vi "rotateAroundModule.vi"(9 "module":u16(ring) items=["Front Left", "Front Right", "Back Left", "Back RIght"], 10 "rotation":dbl) -> ()   [LabVIEW 2020]
uses:
  <vilib>/Rock Robotics/WPI/ThirdParty/REV Robotics/REVLib/Typedef/Spark MAX Control Type.ctl
  <vilib>/Rock Robotics/WPI/ThirdParty/Sensors/navX/_TypeDefs/FRIC_navX_DeviceNumbersTypeDef.ctl
  Robot Global Data.vi
panel:
  # "handy dandy table"
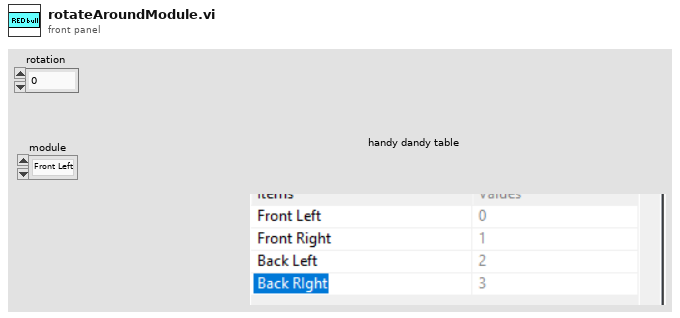
[diagram p1: front panel]
types:
  T1 = typedef "FRIC_navX_DeviceNumbersTypeDef.ctl" = enum16{"Dev0", "Dev1", "Dev2", "Dev3"}
  T2 = typedef "Spark MAX Control Type.ctl" = enum16{"Percent VBus", "Voltage", "Velocity", "Position", "Smart Motion", "Current", "Smart Velocity"}
  T3 = cluster{"Yaw":dbl, "Roll":dbl, "Pitch":dbl, "Heading":dbl, "Fused Heading":dbl}
  T4 = cluster{"FL":cluster{"proportional gain (Kc)":dbl, "integral time (Ti, min)":dbl, "derivative time (Td, min)":dbl}, "FR":cluster{"proportional gain (Kc)":dbl, "integral time (Ti, min)":dbl, "derivative time (Td, min)":dbl}, "BL":cluster{"proportional gain (Kc)":dbl, "integral time (Ti, min)":dbl, "derivative time (Td, min)":dbl}, "BR":cluster{"proportional gain (Kc)":dbl, "integral time (Ti, min)":dbl, "derivative time (Td, min)":dbl}}
  T5 = typedef "WPI_MotorControlDeviceRef.ctl" = cluster{"DeviceStatus":errorcluster, "Type":T6, "PWM":cluster{"PWM Channel":T7, "DeadBand":T8}, "CAN":cluster{"Device Number":u8, "SetOutput VI Ref":variant, "GetOutput VI Ref":variant, "Enable VI Ref":variant, "Disable VI Ref":variant, "Data":variant}, "Invert":bool, "DIO PWM":cluster{"PWM \"Enable\" Channel":T7, "DIOChannel":T9, "PWM Rate":dbl}}
  T6 = typedef "WPI_MotorControlType.ctl" = enum16{"PWM", "CAN", "DIO PWM"}
  T7 = typedef "FPGA_DIOPWMChannel.ctl" = enum8{"PWM 0", "PWM 1", "PWM 2", "PWM 3", "PWM 4", "PWM 5", "PWM 6", "PWM 7", "PWM 8", "PWM 9", "PWM MXP 0", "PWM MXP 1", "PWM MXP 2", "PWM MXP 3", "PWM MXP 4", "PWM MXP 5", "PWM MXP 6", "PWM MXP 7", "PWM MXP 8", "PWM MXP 9", "Invalid"}
  T8 = typedef "WPI_PWMDeadband.ctl" = cluster{"Name":string, "maxPositivePwm":i32, "minPositivePwm":i32, "centerPwm":i32, "maxNegativePwm":i32, "minNegativePwm":i32, "angularRange":u16}
  T9 = typedef "FPGA_DIOChannel.ctl" = enum8{"DIO 0", "DIO 1", "DIO 2", "DIO 3", "DIO 4", "DIO 5", "DIO 6", "DIO 7", "DIO 8", "DIO 9", "DIO MXP 0", "DIO MXP 1", "DIO MXP 2", "DIO MXP 3", "DIO MXP 4", "DIO MXP 5", "DIO MXP 6", "DIO MXP 7", "DIO MXP 8", "DIO MXP 9", "DIO MXP 10", "DIO MXP 11", "DIO MXP 12", "DIO MXP 13", "DIO MXP 14", "DIO MXP 15", "SPI Port CS1", "SPI Port CS2", "SPI Port CS3", "SPI Port MISO", "SPI Port MOSI", "Invalid"}
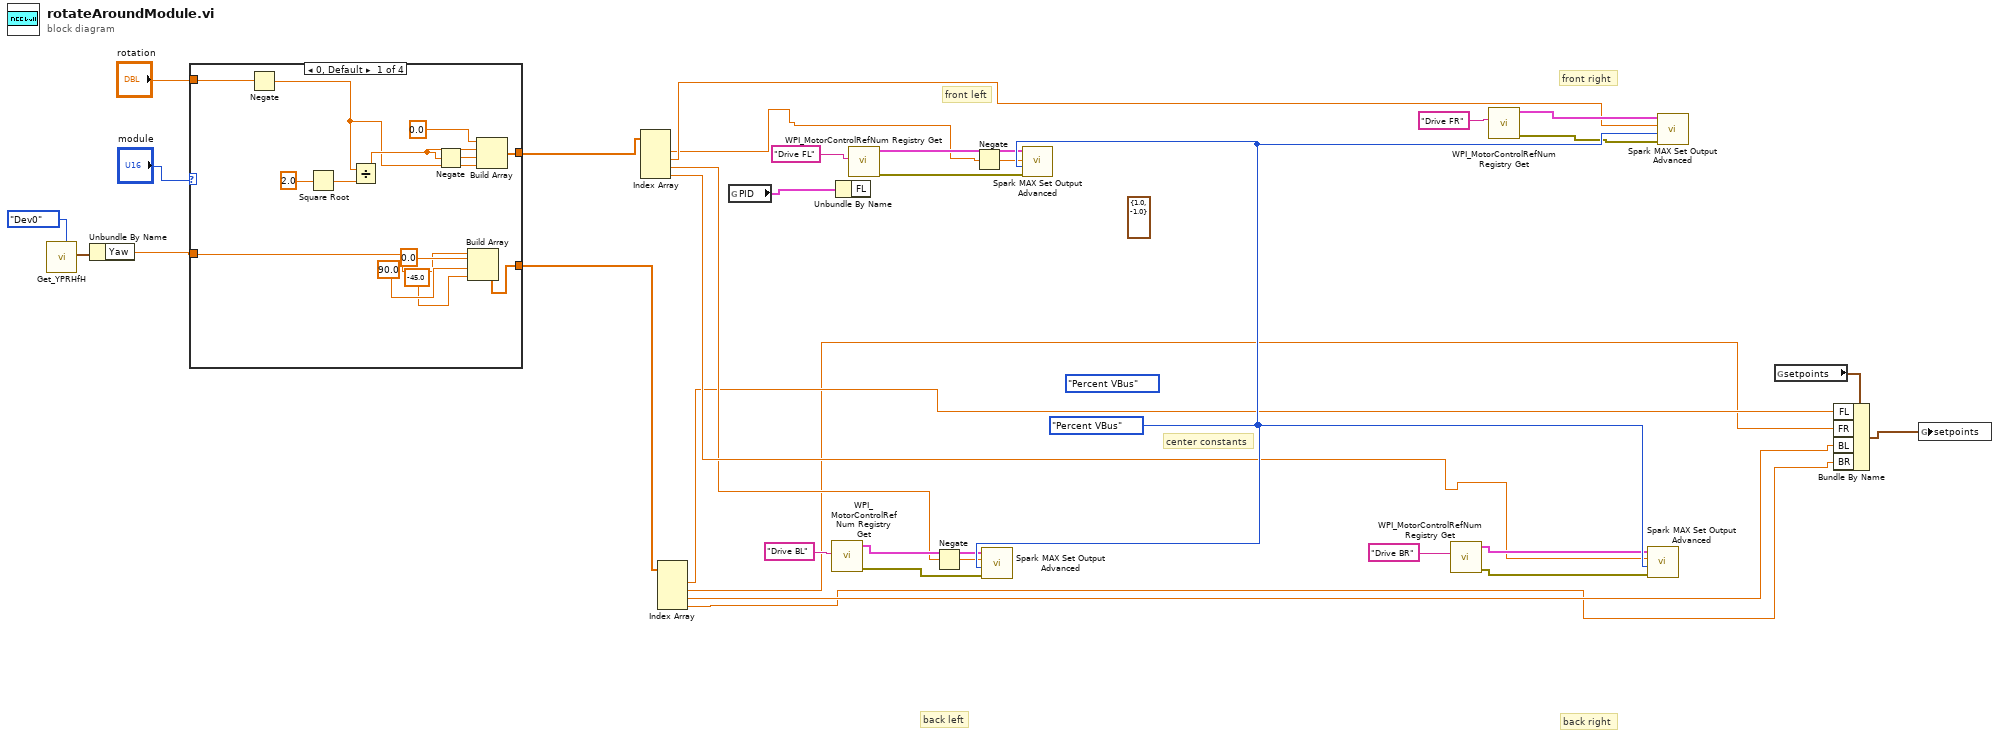
[diagram p0: block diagram]
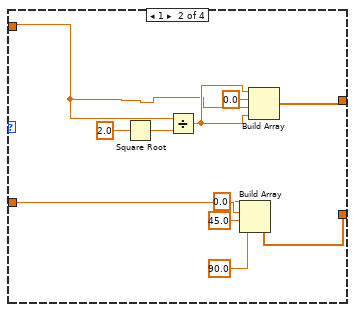
[diagram p2: hidden frame]
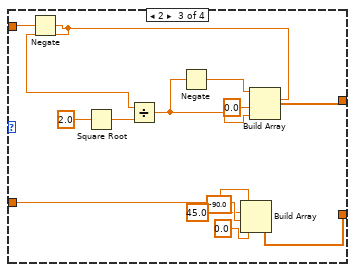
[diagram p3: hidden frame]
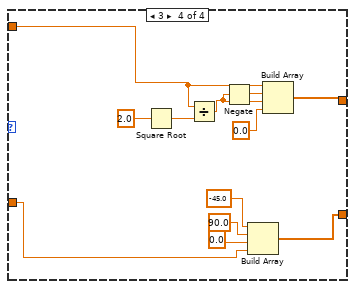
[diagram p4: hidden frame]
diagram:
  w28 = Spark_MAX_Control_Type."Percent VBus" ("Control Mode")
  (unwired) Spark_MAX_Control_Type."Percent VBus" ("Control Mode")
  (unwired) cluster{"output high":dbl, "output low":dbl} {"output high"=1.0, "output low"=-1.0} ("output range")
  # "center constants"
  # "back right"
  # "back left"
  # "front right"
  # "front left"
  n1 = call <vilib>:"Get_YPRHfH.vi"("Device Number"=FRIC_navX_DeviceNumbersTypeDef."Dev0") -> ("YRPHfH"=w12:T3)  [unwired: 10 in]
  n2 = Unbundle By Name(w12) -> ("Yaw"=w7:dbl)
  n3 = case shown="0, Default" "module" {
    tunnel: "rotation" -> [w35 w47 w58 w76]
    tunnel: [w43 w57 w70 w79] -> w17
    tunnel: [w42 w56 w69 w80] -> w14
    tunnel: w7 -> [w38 w55 w68 w81]
    frame 0, Default {
      n4 = Negate(x=w35) -> (-x=w34:dbl)
      n5 = Square Root(x=2.0) -> (sqrt(x)=w45:dbl)
      n6 = Divide(x=w34, y=w45) -> (x/y=w36:dbl)
      n7 = Negate(x=w36) -> (-x=w37:dbl)
      n8 = Build Array(w38, 0.0 ("element"), 90.0 ("element"), -45.0 ("element")) -> (w42:dbl[])
      n9 = Build Array(0.0, w36, w37, w34) -> (w43:dbl[])
    }
    frame 1 {
      n10 = Square Root(x=2.0) -> (sqrt(x)=w53:dbl)
      n11 = Divide(x=w47, y=w53) -> (x/y=w52:dbl)
      n12 = Build Array(0.0 ("element"), w55, 45.0 ("element"), 90.0 ("element")) -> (w56:dbl[])
      n13 = Build Array(w52, 0.0 ("element"), w47, w52) -> (w57:dbl[])
    }
    frame 2 {
      n14 = Negate(x=w58) -> (-x=w59:dbl)
      n15 = Square Root(x=2.0) -> (sqrt(x)=w66:dbl)
      n16 = Divide(x=w59, y=w66) -> (x/y=w61:dbl)
      n17 = Negate(x=w61) -> (-x=w60:dbl)
      n18 = Build Array(-90.0 ("element"), 45.0 ("element"), w68, 0.0 ("element")) -> (w69:dbl[])
      n19 = Build Array(w60, w59, 0.0 ("element"), w61) -> (w70:dbl[])
    }
    frame 3 {
      n20 = Square Root(x=2.0) -> (sqrt(x)=w78:dbl)
      n21 = Divide(x=w76, y=w78) -> (x/y=w71:dbl)
      n22 = Negate(x=w71) -> (-x=w72:dbl)
      n23 = Build Array(-45.0 ("element"), 90.0 ("element"), 0.0 ("element"), w81) -> (w80:dbl[])
      n24 = Build Array(w76, w72, w71, 0.0 ("element")) -> (w79:dbl[])
    }
  }
  n25 = Index Array(array=w17) -> (element #1=w11:dbl, element #2=w16:dbl, element #3=w9:dbl, element #4=w15:dbl)  [unwired: 4 in]
  n26 = Index Array(array=w14) -> (element #1=w4:dbl, element #2=w3:dbl, element #3=w2:dbl, element #4=w1:dbl)  [unwired: 4 in]
  n27 = global read "Robot Global Data.vi" "PID"() -> (w19:T4)
  n28 = call <vilib>:"WPI_MotorControlRefNum Registry Get.vi"("refnum name"="Drive BL") -> ("error out"=w26:errorcluster, "MotorControlDevRef"=w27:T5)  [unwired: 9 in]
  n29 = Unbundle By Name(w19) -> ()  [unwired: 1 out]
  n30 = call <vilib>:"WPI_MotorControlRefNum Registry Get.vi"("refnum name"="Drive FL") -> ("error out"=w24:errorcluster, "MotorControlDevRef"=w25:T5)  [unwired: 9 in]
  n31 = Negate(x=w9) -> (-x=w8:dbl)
  n32 = Negate(x=w11) -> (-x=w10:dbl)
  n33 = call <vilib>:"Spark MAX Set Output Advanced.vi"("error in (no error)"=w26, "Control Mode"=w28, "Setpoint"=w8, "MotorControlDevRef"=w27) -> ()  [unwired: 6 in, 2 out]
  n34 = call <vilib>:"Spark MAX Set Output Advanced.vi"("error in (no error)"=w24, "Control Mode"=w28, "Setpoint"=w10, "MotorControlDevRef"=w25) -> ()  [unwired: 6 in, 2 out]
  n35 = call <vilib>:"WPI_MotorControlRefNum Registry Get.vi"("refnum name"="Drive BR") -> ("error out"=w20:errorcluster, "MotorControlDevRef"=w21:T5)  [unwired: 9 in]
  n36 = call <vilib>:"WPI_MotorControlRefNum Registry Get.vi"("refnum name"="Drive FR") -> ("error out"=w22:errorcluster, "MotorControlDevRef"=w23:T5)  [unwired: 9 in]
  n37 = call <vilib>:"Spark MAX Set Output Advanced.vi"("error in (no error)"=w20, "Control Mode"=w28, "Setpoint"=w15, "MotorControlDevRef"=w21) -> ()  [unwired: 6 in, 2 out]
  n38 = call <vilib>:"Spark MAX Set Output Advanced.vi"("error in (no error)"=w22, "Control Mode"=w28, "Setpoint"=w16, "MotorControlDevRef"=w23) -> ()  [unwired: 6 in, 2 out]
  n39 = global read "Robot Global Data.vi" "setpoints"() -> (w6:cluster{"FL":dbl, "FR":dbl, "BL":dbl, "BR":dbl})
  n40 = Bundle By Name(cluster=w6, "FL"=w4, "FR"=w3, "BL"=w2, "BR"=w1) -> (w5:cluster{"FL":dbl, "FR":dbl, "BL":dbl, "BR":dbl})
  n41 = global write "Robot Global Data.vi" "setpoints"(w5) -> ()
